vi "Hardware Config.vi"() -> ()   [LabVIEW 2022 SP3]
uses:
  Controls/Config.ctl
panel:
  in  "Signal list":bool
  out "Config":T1={"AO config"=[], "AI config"=[], "DI config"=[], "DO config"=[], "TC config"=[{"Channel_Name"="", "Channel_Number"="", "Pre_Scale_min"=0.0, "Pre_Scale_max"=0.0, "units"=4, " type"=7}], "ACC config"=[], "SG config"=[], "Strain Gauge Settings"={"poisson ratio"=0.3, "nominal gage resistance"=120.0, "gage factor"=2.08}, "Bridge Settings"={"voltage excitation value"=3.3, "voltage excitation source"=10200, "initial bridge voltage"=0.0, "lead wire resistance"=1.7, "strain configuration"=10271}, "Sample Rate"={"AI Sample Rate"=[], "AO Sample Rate"=[], "DI Sample Rate"=[], "TC Sample Rate"=[], "DO Sample Rate"=[], "SG Sample Rate"=[], "ACC Sample Rate"=[]}} {"Bridge Settings"."strain configuration" items=["Full Bridge I"=10183, "Full Bridge II"=10184, "Full Bridge III"=10185, "Half Bridge I"=10188, "Half Bridge II"=10189, "Quarter Bridge I"=10271, "Quarter Bridge II"=10272]; "Bridge Settings"."voltage excitation source" items=["Internal"=10200, "External"=10167, "None"=10230]; "ACC config"."Terminal configuration" items=["default"=-1, "RSE"=10083, "NRSE"=10078, "Differential"=10106, "Pseudodifferential"=12529]; "ACC config"."Sensitivity units" items=["mVolts/g"=12509, "Volts/g"=12510]; "TC config"."type" items=["J"=10072, "K"=10073, "N"=10077, "R"=10082, "S"=10085, "T"=10086, "B"=10047, "E"=10055]; "TC config"."units" items=["Deg C", "Deg F", "Kelvins", "Deg R", "From Custom Scale"]}
  in  "Cancel":bool
  in  "Load Configuration":bool
  in  "New configuration":bool
  in  "Save Config":bool
  in  "Tab Control":T2(tab)
  in  "DO Sample Rate":dbl[](array[numeric]) format="%#_g Hz"
  in  "DO config":T3(array[cluster])=[{"Channel_Name"="", "Channel_Number"="", "Default_Value"=FALSE, "Units"=FALSE}]
  out "DO Device List":string[](array[string])
  in  "DI Sample Rate":dbl[](array[numeric]) format="%#_g Hz"
  in  "DI config":T3(array[cluster])
  out "DI Device List":string[](array[string])
  in  "AO Sample Rate":dbl[](array[numeric]) format="%#_g Hz"
  in  "AO config":T4(array[cluster])
  out "AO Device List":string[](array[string])
  in  "AI Sample Rate":dbl[](array[numeric]) format="%#_g Hz"
  in  "AI config":T5(array[cluster])
  out "AI Device List":string[](array[string])
  in  "TC Sample Rate":dbl[](array[numeric]) format="%#_g Hz"
  in  "TC config":T6(array[cluster]) {"thermocouple type" items=["J", "K", "N", "R", "S", "T", "B", "E"]; "units" items=["Deg C", "Deg F", "Kelvins", "Deg R", "From Custom Scale"]}
  out "TC Device List":string[](array[string])
  in  "ACC Sample Rate":dbl[](array[numeric]) format="%#_g Hz"
  in  "ACC config":T7(array[cluster]) {"Sensitivity units" items=["mVolts/g"=12509, "Volts/g"=12510]; "Terminal configuration" items=["default"=-1, "RSE"=10083, "NRSE"=10078, "Differential"=10106, "Pseudodifferential"=12529]}
  out "ACC Device List":string[](array[string])
  out "SG Device List":string[](array[string])
  in  "SG Sample Rate":dbl[](array[numeric]) format="%#_g Hz"
  in  "SG config":T8(array[cluster])
  in  "SG Settings":T9={"gage factor"=2.08, "nominal gage \nresistance"=120.0, "poisson ratio"=0.3}
  in  "Bridge Settings":T10={"voltage excitation value"=3.3, "voltage excitation source"=10200, "initial bridge voltage"=0.0, "lead wire resistance"=1.7, "strain configuration"=10271} {"strain configuration" items=["Full Bridge I"=10183, "Full Bridge II"=10184, "Full Bridge III"=10185, "Half Bridge I"=10188, "Half Bridge II"=10189, "Quarter Bridge I"=10271, "Quarter Bridge II"=10272]; "voltage excitation source" items=["Internal"=10200, "External"=10167, "None"=10230]}
  # "DO_Channel_Name"
  # "DO_Channel_Number"
  # "Default Value"
  # "Invert?"
  # "DI_Channel_Name"
  # "DI_Channel_Number"
  # "Default Value"
  # "Invert?"
  # "AO_Channel_Name"
  # "AO_Channel_Number"
  # "Default Value"
  # "Units"
  # "AI_Channel_Name"
  # "AI_Channel_Number"
  # "Pre_Scale_min"
  # "Pre_Scale_max"
  # "Scale_min"
  # "Scale_max"
  # "Units"
  # "TC_Channel_Name"
  # "TC_Channel_Number"
  # "Max_Value"
  # "Units"
  # "Type"
  # "Min_Value"
  # "ACC_Channel_Name"
  # "ACC_Channel_Number"
  # "Min_Value"
  # "Max_Value"
  # "Terminal Config"
  # "Sensitivity"
  # "Sensitivity Units"
  # "SG_Channel_Name"
  # "SG_Channel_Number"
  # "Min_Value"
  # "Max_Value"
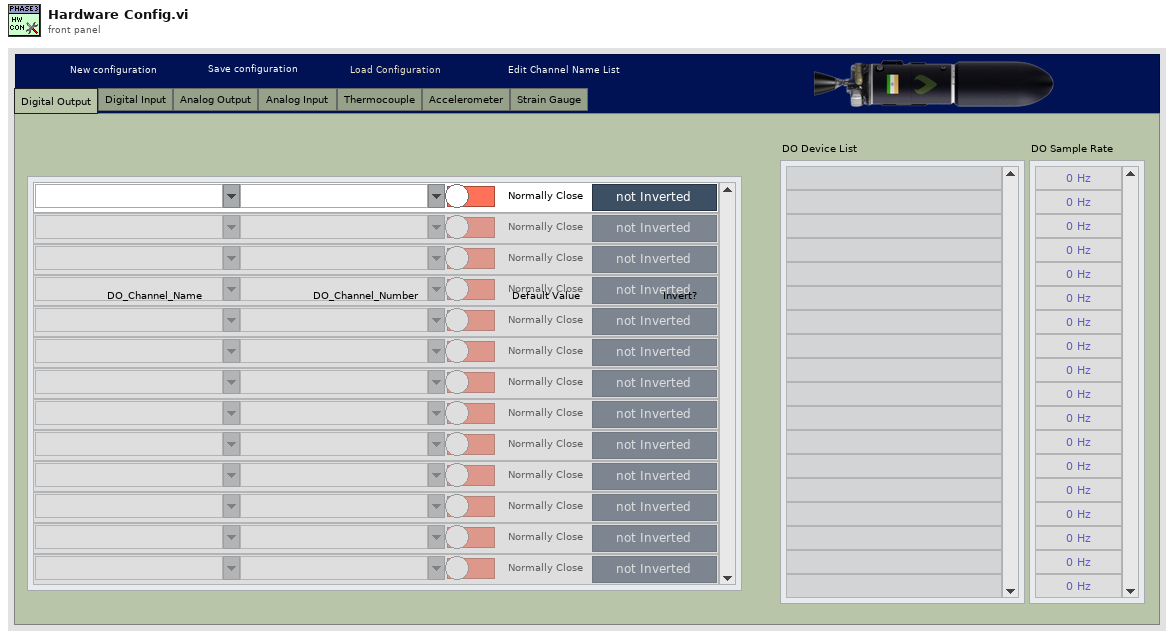
[diagram p1: front panel]
types:
  T1 = typedef "Config.ctl" = cluster{"AO config":cluster{"Channel_Name":string, "Channel_Number":string, "Default_Value":dbl, "Units":string}[], "AI config":cluster{"Channel_Name":string, "Channel_Number":string, "Pre_Scale_min":dbl, "Pre_Scale_max":dbl, "Sensor_min":dbl, "Sensor_max":dbl, "Units":string}[], "DI config":cluster{"Channel_Name":string, "Channel_Number":string, "Default_Value":bool, "DI invert?":bool}[], "DO config":cluster{"Channel_Name":string, "Channel_Number":string, "Default_Value":bool, "DO invert?":bool}[], "TC config":cluster{"Channel_Name":string, "Channel_Number":string, "Pre_Scale_min":dbl, "Pre_Scale_max":dbl, "units":i32, " type":i32}[], "ACC config":cluster{"Channel_Name":string, "Channel_Number":string, "Pre_Scale_min":dbl, "Pre_Scale_max":dbl, "Terminal configuration":i32, "Sensitivity":dbl, "Sensitivity units":i32}[], "SG config":cluster{"Channel_Name":string, "Channel_Number":string, "Pre_Scale_min":dbl, "Pre_Scale_max":dbl}[], "Strain Gauge Settings":cluster{"poisson ratio":dbl, "nominal gage resistance":dbl, "gage factor":dbl}, "Bridge Settings":cluster{"voltage excitation value":dbl, "voltage excitation source":i32, "initial bridge voltage":dbl, "lead wire resistance":dbl, "strain configuration":i32}, "Sample Rate":cluster{"AI Sample Rate":dbl[], "AO Sample Rate":dbl[], "DI Sample Rate":dbl[], "TC Sample Rate":dbl[], "DO Sample Rate":dbl[], "SG Sample Rate":dbl[], "ACC Sample Rate":dbl[]}}
  T2 = enum32{"Digital Output", "Digital Input", "Analog Output", "Analog Input ", "Thermocouple", "Accelerometer", "Strain Gauge"}
  T3 = cluster{"Channel_Name":string, "Channel_Number":string, "Default_Value":bool, "Units":bool}[]
  T4 = cluster{"Channel_Name":string, "Channel_Number":string, "Default_Value":dbl, "Units":string}[]
  T5 = cluster{"Channel_Name":string, "Channel_Number":string, "Pre_Scale_min":dbl, "Pre_Scale_max":dbl, "Sensor_min":dbl, "Sensor_max":dbl, "Units":string}[]
  T6 = cluster{"Channel_Name":string, "Channel_Number":string, "Pre_Scale_min":dbl, "Pre_Scale_max":dbl, "units":i32, "thermocouple type":i32}[]
  T7 = cluster{"Channel_Name":string, "Channel_Number":string, "Pre_Scale_min":dbl, "Pre_Scale_max":dbl, "Terminal configuration":i32, "Sensitivity":dbl, "Sensitivity units":i32}[]
  T8 = cluster{"Channel_Name":string, "Channel_Number":string, "Pre_Scale_min":dbl, "Pre_Scale_max":dbl}[]
  T9 = cluster{"gage factor":dbl, "nominal gage \nresistance":dbl, "poisson ratio":dbl}
  T10 = cluster{"voltage excitation value":dbl, "voltage excitation source":i32, "initial bridge voltage":dbl, "lead wire resistance":dbl, "strain configuration":i32}
  T11 = cluster{"Data":T1, "path":path, "Name ref":refnum<vi>[], "Names":string[][], "Signal path":path, "SR":cluster{"AI Sample Rate":dbl[], "AO Sample Rate":dbl[], "DI Sample Rate":dbl[], "TC Sample Rate":dbl[], "DO Sample Rate":dbl[], "SG Sample Rate":dbl[], "ACC Sample Rate":dbl[]}, "Device List":cluster{"AO Cards":tag[], "AI Cards":tag[], "DI Cards":tag[], "DO Cards":tag[]}}
  T12 = typedef "file folder ctl.ctl" = cluster{"Datalog path":path, "Configuration path":path, "Signal list path":path, "Sub vi's":path, "Authentication":path}
  T13 = cluster{"AI":string[], "DI":string[], "DO":string[], "SG":string[], "AO":string[], "TC":string[], "ACC":string[]}
  T14 = cluster{"AO Cards":tag[], "AI Cards":tag[], "DI Cards":tag[], "DO Cards":tag[]}
  T15 = cluster{"AI Channel list":tag[], "AO Channel list":tag[], "DO Channel list ":tag[], "DI Channel list":tag[]}
  T16 = cluster{"AI Sample Rate":dbl[], "AO Sample Rate":dbl[], "DI Sample Rate":dbl[], "TC Sample Rate":dbl[], "DO Sample Rate":dbl[], "SG Sample Rate":dbl[], "ACC Sample Rate":dbl[]}
  T17 = enum16{"open", "replace", "create", "open or create", "replace or create", "replace or create with confirmation"}
  T18 = enum32{"Invalid", "Standard", "Closed", "Hidden", "Minimized", "Maximized"}
  T19 = cluster{"Channel_Name":string, "Channel_Number":string, "Default_Value":bool, "DI invert?":bool}[]
  T20 = cluster{"Channel_Name":string, "Channel_Number":string, "Default_Value":bool, "DO invert?":bool}[]
  T21 = cluster{"Channel_Name":string, "Channel_Number":string, "Pre_Scale_min":dbl, "Pre_Scale_max":dbl, "units":i32, " type":i32}[]
  T22 = cluster{"poisson ratio":dbl, "nominal gage resistance":dbl, "gage factor":dbl}
  T23 = cluster{"Channel_Name":string, "Channel_Number":string}
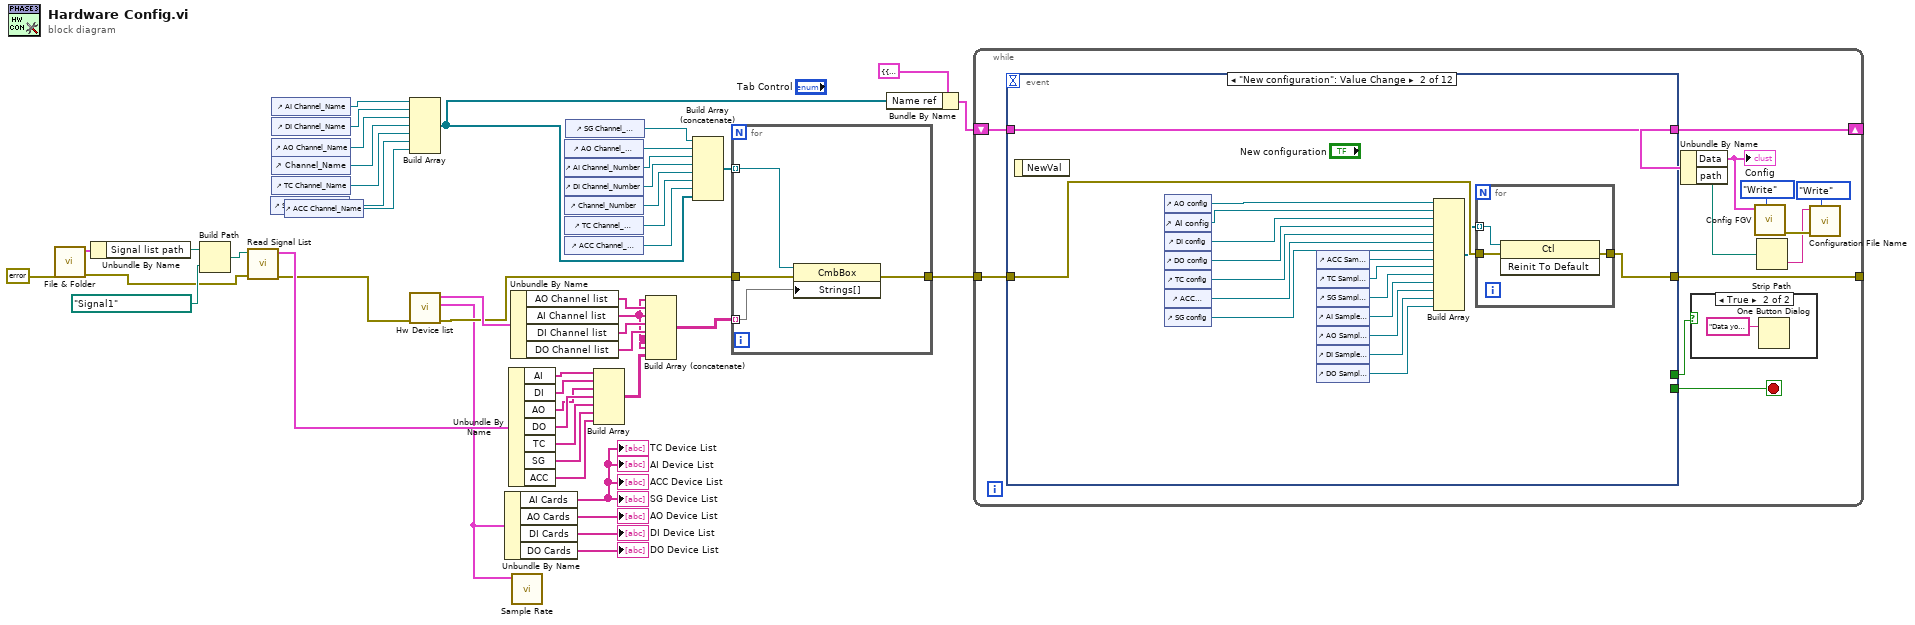
[diagram p0: block diagram]
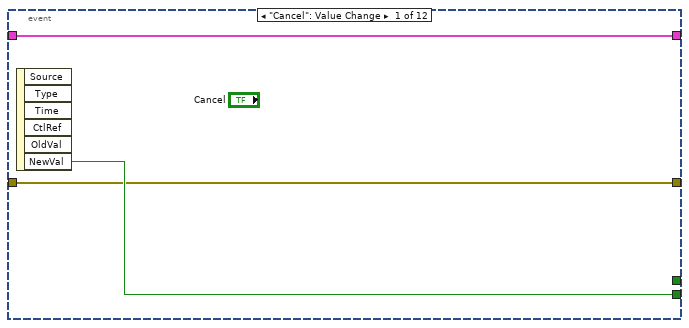
[diagram p3: hidden frame]
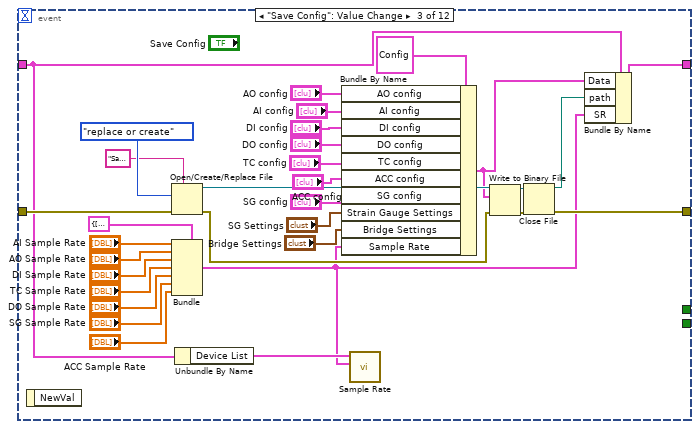
[diagram p4: hidden frame]
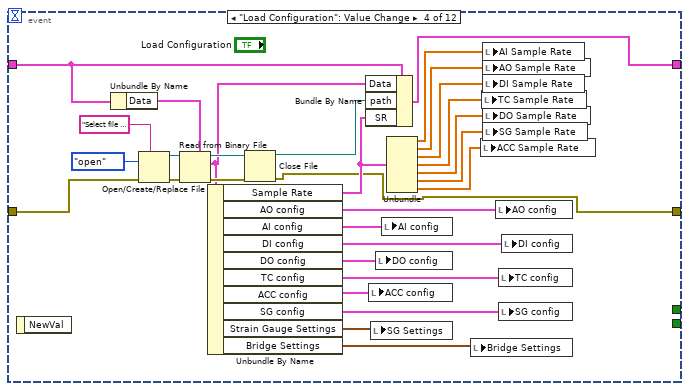
[diagram p5: hidden frame]
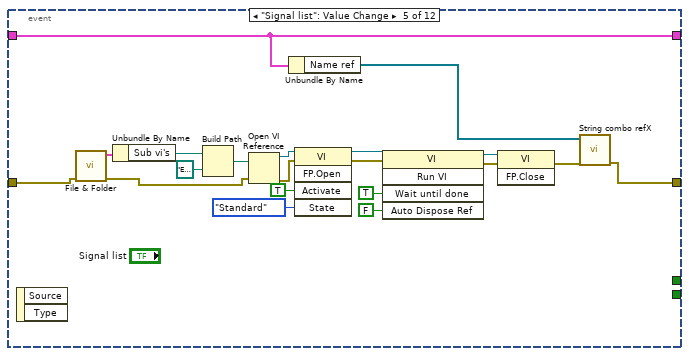
[diagram p6: hidden frame]
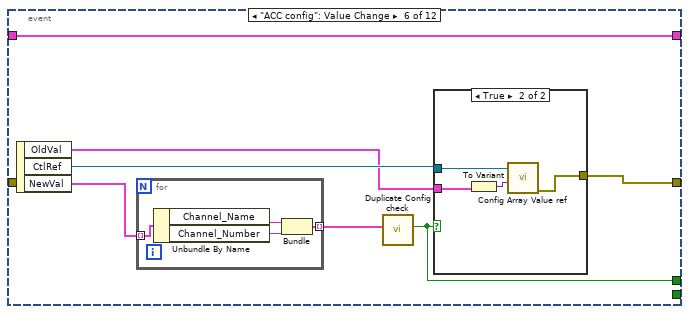
[diagram p7: hidden frame]
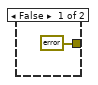
[diagram p8: hidden frame]
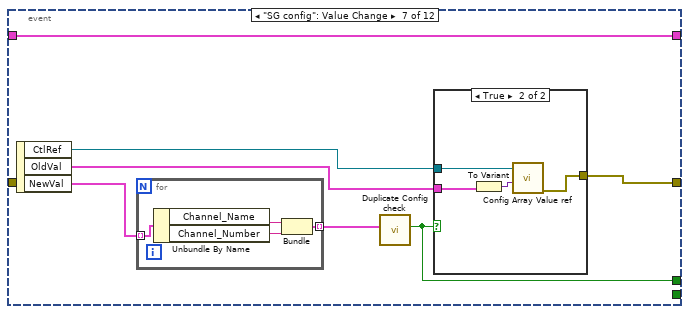
[diagram p9: hidden frame]
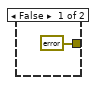
[diagram p10: hidden frame]
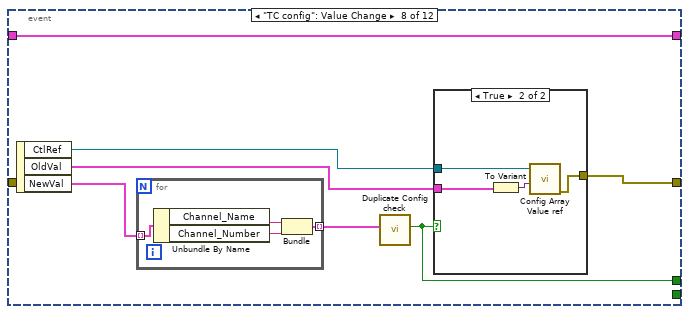
[diagram p11: hidden frame]
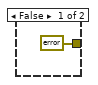
[diagram p12: hidden frame]
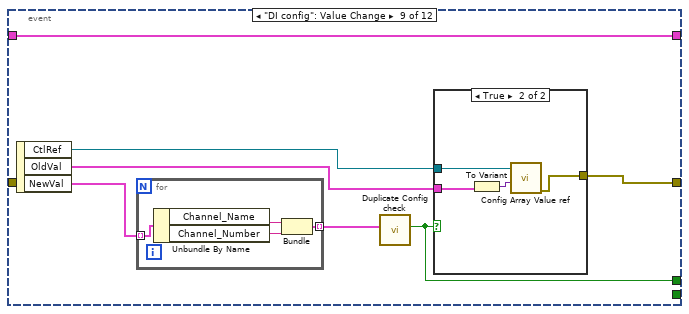
[diagram p13: hidden frame]
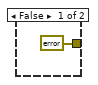
[diagram p14: hidden frame]
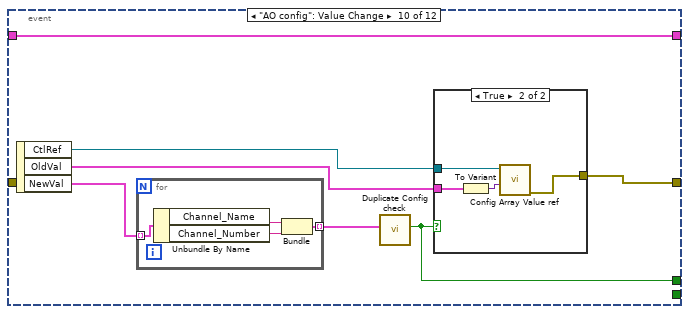
[diagram p15: hidden frame]
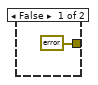
[diagram p16: hidden frame]
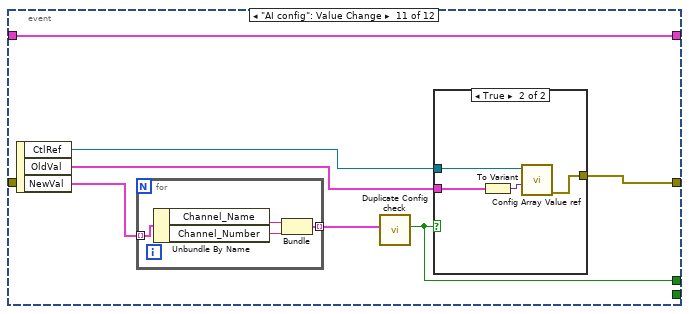
[diagram p17: hidden frame]
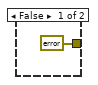
[diagram p18: hidden frame]
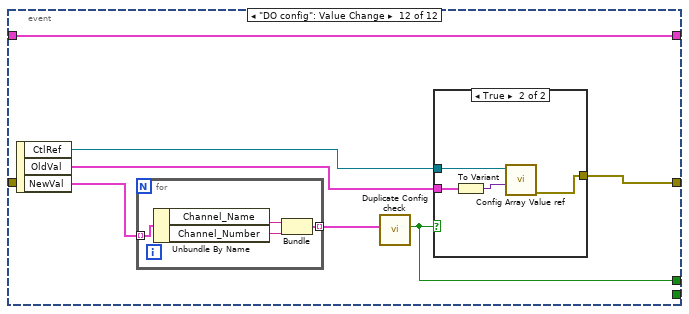
[diagram p19: hidden frame]
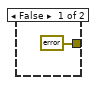
[diagram p20: hidden frame]
diagram:
  n1 = call "File & Folder.vi"("error in (no error)"=errorcluster {"status"=FALSE, "code"=0, "source"=""} ("error in")) -> ("error out"=w24:errorcluster, "File Output"=w30:T12)  [unwired: 9 in]
  n2 = Unbundle By Name(w30) -> ("Signal list path"=w29:path)
  n3 = Build Path(base path=w29, name or relative path=path "Signal1") -> (appended path=w1:path)
  n4 = call "Read Signal List.vi"("error in"=w24, "file path (use dialog)"=w1) -> ("error out"=w4:errorcluster, "Names"=w23:T13)  [unwired: 8 in]
  n5 = control-ref of="SG Channel_Name"() -> (w9:refnum<vi>)
  n6 = control-ref of="AI Channel_Name"() -> (w27:refnum<vi>)
  n7 = control-ref of="DI Channel_Name"() -> (w26:refnum<vi>)
  n8 = control-ref of="AO Channel_Name"() -> (w11:refnum<vi>)
  n9 = control-ref of="Channel_Name"() -> (w10:refnum<vi>)
  n10 = control-ref of="TC Channel_Name"() -> (w25:refnum<vi>)
  n11 = control-ref of="ACC Channel_Name"() -> (w8:refnum<vi>)
  n12 = Build Array(w27, w26, w11, w10, w25, w9, w8) -> (w12:refnum<vi>[])
  n13 = call "Hw Device list.vi"("error in (no error)"=w4) -> ("error out"=w38:errorcluster, "Device List"=w2:T14, "Channel List"=w39:T15)  [unwired: 8 in]
  n14 = Unbundle By Name(w2) -> ("AI Cards"=→"AI Device List" →"TC Device List" →"ACC Device List" →"SG Device List":tag[], "AO Cards"=→"AO Device List":tag[], "DI Cards"=→"DI Device List":tag[], "DO Cards"=→"DO Device List":tag[])
  n15 = Unbundle By Name(w23) -> ("AI"=w22:string[], "DI"=w21:string[], "AO"=w16:string[], "DO"=w20:string[], "TC"=w19:string[], "SG"=w18:string[], "ACC"=w17:string[])
  n16 = Unbundle By Name(w39) -> ("AO Channel list"=w33:tag[], "AI Channel list"=w32:tag[], "DI Channel list"=w42:tag[], "DO Channel list"=w41:tag[])
  n17 = call "Sample Rate.vi"("Device List"=w2) -> ()  [unwired: 11 in]
  n18 = control-ref of="AO Channel_Number"() -> (w47:refnum<vi>)
  n19 = control-ref of="AI Channel_Number"() -> (w46:refnum<vi>)
  n20 = control-ref of="DI Channel_Number"() -> (w45:refnum<vi>)
  n21 = control-ref of="Channel_Number"() -> (w44:refnum<vi>)
  n22 = control-ref of="TC Channel_Number"() -> (w36:refnum<vi>)
  n23 = control-ref of="ACC Channel_Number"() -> (w35:refnum<vi>)
  n24 = control-ref of="SG Channel_Number"() -> (w34:refnum<vi>)
  n25 = Build Array(w22, w21, w16, w20, w19, w18, w17) -> (w15:string[][])
  n26 = Build Array (concatenate)(w32, w33, w32, w42, w41, w32, w32, w15) -> (w40:string[][])
  n27 = Build Array (concatenate)(w34, w47, w46, w45, w44, w36, w35, w12) -> (w43:refnum<vi>[])
  n28 = for {
    tunnel: w43 -> [w51] mode=indexing
    tunnel: w40 -> [w48] mode=indexing
    tunnel: [w50] -> w37
    tunnel: w38 -> [w49]
    n29 = property class="CmbBox"(reference=w51, error in=w49, "Strings[]"=w48) -> (error out=w50:errorcluster)  [unwired: 1 out]
  }
  n30 = Bundle By Name(cluster=T11 {"Data"={"AO config"=[], "AI config"=[], "DI config"=[], "DO config"=[], "TC config"=[{"Channel_Name"="", "Channel_Number"="", "Pre_Scale_min"=0.0, "Pre_Scale_max"=0.0, "units"=4, " type"=7}], "ACC config"=[], "SG config"=[], "Strain Gauge Settings"={"poisson ratio"=0.3, "nominal gage resistance"=120.0, "gage factor"=2.08}, "Bridge Settings"={"voltage excitation value"=3.3, "voltage excitation source"=10200, "initial bridge voltage"=0.0, "lead wire resistance"=1.7, "strain configuration"=10271}, "Sample Rate"={"AI Sample Rate"=[], "AO Sample Rate"=[], "DI Sample Rate"=[], "TC Sample Rate"=[], "DO Sample Rate"=[], "SG Sample Rate"=[], "ACC Sample Rate"=[]}}, "path"=path "", "Name ref"=[], "Names"=[], "Signal path"=path "", "SR"={"AI Sample Rate"=[], "AO Sample Rate"=[], "DI Sample Rate"=[], "TC Sample Rate"=[], "DO Sample Rate"=[], "SG Sample Rate"=[], "ACC Sample Rate"=[]}, "Device List"={"AO Cards"=["PXI1Slot2"], "AI Cards"=["cDAQ1Mod1", "cDAQ1Mod2", "cDAQ1Mod3", "cDAQ1Mod4"], "DI Cards"=["cDAQ1Mod5", "PXI1Slot2", "PXI1Slot3"], "DO Cards"=["cDAQ1Mod5", "PXI1Slot2", "PXI1Slot3"]}}, "Name ref"=w12) -> (w14:T11)
  n31 = while {
    shift-right: [w59] -> _
    shift-left: w14 -> [w60]
    tunnel: w37 -> [w62]
    tunnel: [w61] -> _
    stop <- w63 stop-if-true
    n32 = event shown="[1] \"New configuration\": Value Change" {
      selector: _ -> [_ _ _ _ _ _ _ _ _ _ _ _]
      dyn-events: _ -> [_ _ _ _ _ _ _ _ _ _ _ _]
      timeout: _ -> [_ _ _ _ _ _ _ _ _ _ _ _]
      tunnel: [w66 _ _ _ _ _ _ _ _ _ _ _] -> w63
      tunnel: w62 -> [w65 w85 w120 w150 w170 _ _ _ _ _ _ _]
      tunnel: [w65 w84 w116 w127 w152 w172 w190 w206 w222 w238 w254 w270] -> w61
      tunnel: w60 -> [w67 w83 w91 w141 w155 w177 w193 w209 w225 w241 w257 w273]
      tunnel: [w67 w83 w108 w142 w155 w177 w193 w209 w225 w241 w257 w273] -> w59
      tunnel: [_ _ _ _ _ w171 w187 w203 w219 w235 w251 w267] -> w55
      event "Cancel": Value Change {
        n33 = event-data() -> ("NewVal"=w66:bool)  [unwired: 1 in, 5 out]
      }
      event "New configuration": Value Change {
        n34 = event-data() -> ()  [unwired: 1 in, 1 out]
        n35 = control-ref of="AO config"() -> (w78:refnum<vi>)
        n36 = control-ref of="AI config"() -> (w79:refnum<vi>)
        n37 = control-ref of="DI config"() -> (w80:refnum<vi>)
        n38 = control-ref of="DO config"() -> (w81:refnum<vi>)
        n39 = control-ref of="TC config"() -> (w77:refnum<vi>)
        n40 = control-ref of="ACC config"() -> (w76:refnum<vi>)
        n41 = control-ref of="SG config"() -> (w75:refnum<vi>)
        n42 = control-ref of="ACC Sample Rate"() -> (w74:refnum<vi>)
        n43 = control-ref of="TC Sample Rate"() -> (w73:refnum<vi>)
        n44 = control-ref of="SG Sample Rate"() -> (w72:refnum<vi>)
        n45 = control-ref of="AI Sample Rate"() -> (w71:refnum<vi>)
        n46 = control-ref of="AO Sample Rate"() -> (w70:refnum<vi>)
        n47 = control-ref of="DI Sample Rate"() -> (w69:refnum<vi>)
        n48 = control-ref of="DO Sample Rate"() -> (w68:refnum<vi>)
        n49 = Build Array(w78, w79, w80, w81, w77, w76, w75, w74, w73, w72, w71, w70, w69, w68) -> (w82:refnum<vi>[])
        n50 = for {
          tunnel: w82 -> [w88] mode=indexing
          tunnel: w85 -> [w87]
          tunnel: [w86] -> w84
          n51 = invoke class="Ctl" method="Reinit To Default"(reference=w88, error in=w87) -> (error out=w86:errorcluster)  [unwired: 1 in, 2 out]
        }
      }
      event "Save Config": Value Change {
        n52 = event-data() -> ()  [unwired: 1 in, 1 out]
        n53 = Open/Create/Replace File(error in=w120, prompt="Save Changes", operation (0:open)=T17."replace or create") -> (refnum out=w115:refnum<file>, error out=w119:errorcluster)  [unwired: 3 in, 1 out]
        n54 = Bundle(cluster=T16 {"AI Sample Rate"=[], "AO Sample Rate"=[], "DI Sample Rate"=[], "TC Sample Rate"=[], "DO Sample Rate"=[], "SG Sample Rate"=[], "ACC Sample Rate"=[]} ("Sample Rate"), "AI Sample Rate"="AI Sample Rate", "AO Sample Rate"="AO Sample Rate", "DI Sample Rate"="DI Sample Rate", "TC Sample Rate"="TC Sample Rate", "DO Sample Rate"="DO Sample Rate", "SG Sample Rate"="SG Sample Rate", "ACC Sample Rate"="ACC Sample Rate") -> (w89:T16)
        n55 = Unbundle By Name(w91) -> ("Device List"=w90:T14)
        n56 = Bundle By Name(cluster=T1 {"AO config"=[], "AI config"=[], "DI config"=[], "DO config"=[], "TC config"=[{"Channel_Name"="", "Channel_Number"="", "Pre_Scale_min"=0.0, "Pre_Scale_max"=0.0, "units"=4, " type"=7}], "ACC config"=[], "SG config"=[], "Strain Gauge Settings"={"poisson ratio"=0.3, "nominal gage resistance"=120.0, "gage factor"=2.08}, "Bridge Settings"={"voltage excitation value"=3.3, "voltage excitation source"=10200, "initial bridge voltage"=0.0, "lead wire resistance"=1.7, "strain configuration"=10271}, "Sample Rate"={"AI Sample Rate"=[], "AO Sample Rate"=[], "DI Sample Rate"=[], "TC Sample Rate"=[], "DO Sample Rate"=[], "SG Sample Rate"=[], "ACC Sample Rate"=[]}} ("Data"), "AO config"="AO config", "AI config"="AI config", "DI config"="DI config", "DO config"="DO config", "TC config"="TC config", "ACC config"="ACC config", "SG config"="SG config", "Strain Gauge Settings"="SG Settings", "Bridge Settings"="Bridge Settings", "Sample Rate"=w89) -> (w106:T1)
        n57 = call "Sample Rate.vi"("Sample Rate"=w89, "Device List"=w90) -> ()  [unwired: 10 in]
        n58 = Write to Binary File(file (use dialog)=w115, data=w106, error in=w119) -> (refnum out=w118:refnum<file>, error out=w117:errorcluster)  [unwired: 3 in, 1 out]
        n59 = Close File(refnum=w118, error in=w117) -> (path=w102:path, error out=w116:errorcluster)
        n60 = Bundle By Name(cluster=w91, "Data"=w106, "path"=w102, "SR"=w89) -> (w108:T11)
      }
      event "Load Configuration": Value Change {
        n61 = event-data() -> ()  [unwired: 1 in, 1 out]
        n62 = Unbundle By Name(w141) -> ("Data"=w143:T1)
        n63 = Open/Create/Replace File(error in=w150, prompt="Select file to load", operation (0:open)=T17."open") -> (refnum out=w146:refnum<file>, error out=w149:errorcluster)  [unwired: 3 in, 1 out]
        n64 = Read from Binary File(5:w143, 8:w149, 11:w146) -> (0:w147:errorcluster, 2:w140:T1, 3:w148:refnum<file>)  [unwired: 3 in, 1 out]
        n65 = Unbundle By Name(w140) -> ("Sample Rate"=w129:T16, "AO config"=w139:T4, "AI config"=w138:T5, "DI config"=w137:T19, "DO config"=w136:T20, "TC config"=w135:T21, "ACC config"=w134:T7, "SG config"=w133:T8, "Strain Gauge Settings"=w131:T22, "Bridge Settings"=w130:T10)
        n66 = Close File(refnum=w148, error in=w147) -> (path=w132:path, error out=w127:errorcluster)
        n67 = Bundle By Name(cluster=w141, "Data"=w140, "path"=w132, "SR"=w129) -> (w142:T11)
        n68 = local write "ACC config"(w134) -> ()
        n69 = local write "SG Settings"(w131) -> ()
        n70 = local write "DO config"(w136) -> ()
        n71 = local write "AI config"(w138) -> ()
        n72 = Unbundle(w129) -> ("AI Sample Rate"=w128:dbl[], "AO Sample Rate"=w126:dbl[], "DI Sample Rate"=w125:dbl[], "TC Sample Rate"=w124:dbl[], "DO Sample Rate"=w123:dbl[], "SG Sample Rate"=w122:dbl[], "ACC Sample Rate"=w121:dbl[])
        n73 = local write "Bridge Settings"(w130) -> ()
        n74 = local write "ACC Sample Rate"(w121) -> ()
        n75 = local write "TC Sample Rate"(w124) -> ()
        n76 = local write "AI Sample Rate"(w128) -> ()
        n77 = local write "AO Sample Rate"(w126) -> ()
        n78 = local write "DI Sample Rate"(w125) -> ()
        n79 = local write "DO Sample Rate"(w123) -> ()
        n80 = local write "SG Sample Rate"(w122) -> ()
        n81 = local write "AO config"(w139) -> ()
        n82 = local write "TC config"(w135) -> ()
        n83 = local write "SG config"(w133) -> ()
        n84 = local write "DI config"(w137) -> ()
      }
      event "Signal list": Value Change {
        n85 = event-data() -> ()  [unwired: 1 in, 2 out]
        n86 = call "File & Folder.vi"("error in (no error)"=w170) -> ("error out"=w166:errorcluster, "File Output"=w169:T12)  [unwired: 9 in]
        n87 = Unbundle By Name(w169) -> ("Sub vi's"=w168:path)
        n88 = Build Path(base path=w168, name or relative path=path "Edit Channel Name list.vi") -> (appended path=w151:path)
        n89 = Open VI Reference(vi path=w151, error in (no error)=w166) -> (vi reference=w157:refnum<vi>, error out=w156:errorcluster)  [unwired: 4 in]
        n90 = Unbundle By Name(w155) -> ("Name ref"=w154:refnum<vi>[])
        n91 = invoke class="VI" method="FP.Open"(reference=w157, error in=w156, "Activate"=TRUE ("Activate?"), "State"=T18."Standard") -> (reference out=w165:refnum<vi>, error out=w164:errorcluster)  [unwired: 1 in, 3 out]
        n92 = invoke class="VI" method="Run VI"(reference=w165, error in=w164, "Wait until done"=TRUE ("Wait Until Done"), "Auto Dispose Ref"=FALSE ("Auto Dispose Reference")) -> (reference out=w163:refnum<vi>, error out=w162:errorcluster)  [unwired: 1 in, 3 out]
        n93 = invoke class="VI" method="FP.Close"(reference=w163, error in=w162) -> (error out=w153:errorcluster)  [unwired: 1 in, 2 out]
        n94 = call "String combo refX.vi"("error out"=w153, "Ctrl ref"=w154) -> ("error out 2"=w152:errorcluster)  [unwired: 9 in]
      }
      event "ACC config": Value Change {
        n95 = event-data() -> ("OldVal"=w173:T7, "CtlRef"=w174:refnum<vi>, "NewVal"=w176:T7)  [unwired: 1 in]
        n96 = for {
          tunnel: w176 -> [w181] mode=indexing
          tunnel: [w178] -> w175 mode=indexing
          n97 = Unbundle By Name(w181) -> ("Channel_Name"=w179:string, "Channel_Number"=w180:string)
          n98 = Bundle("Channel_Name"=w179, "Channel_Number"=w180) -> (w178:T23)  [unwired: 1 in]
        }
        n99 = call "Duplicate Config check.vi"("Data in"=w175) -> ("Channel list indication"=w171:bool)  [unwired: 10 in]
        n100 = case shown="True" w171 {
          tunnel: w174 -> [_ w185]
          tunnel: w173 -> [_ w184]
          tunnel: [errorcluster {"status"=FALSE, "code"=0, "source"=""} ("error out") w183] -> w172
          frame False {
          }
          frame True {
            n101 = To Variant(anything=w184) -> (Variant=w186:variant)
            n102 = call "Config Array Value ref.vi"("Value"=w186, "Array in"=w185) -> ("error out"=w183:errorcluster)  [unwired: 9 in]
          }
        }
      }
      event "SG config": Value Change {
        n103 = event-data() -> ("CtlRef"=w189:refnum<vi>, "OldVal"=w188:T8, "NewVal"=w192:T8)  [unwired: 1 in]
        n104 = for {
          tunnel: w192 -> [w197] mode=indexing
          tunnel: [w194] -> w191 mode=indexing
          n105 = Unbundle By Name(w197) -> ("Channel_Name"=w195:string, "Channel_Number"=w196:string)
          n106 = Bundle("Channel_Name"=w195, "Channel_Number"=w196) -> (w194:T23)  [unwired: 1 in]
        }
        n107 = call "Duplicate Config check.vi"("Data in"=w191) -> ("Channel list indication"=w187:bool)  [unwired: 10 in]
        n108 = case shown="True" w187 {
          tunnel: w189 -> [_ w201]
          tunnel: w188 -> [_ w200]
          tunnel: [errorcluster {"status"=FALSE, "code"=0, "source"=""} ("error out") w199] -> w190
          frame False {
          }
          frame True {
            n109 = To Variant(anything=w200) -> (Variant=w202:variant)
            n110 = call "Config Array Value ref.vi"("Value"=w202, "Array in"=w201) -> ("error out"=w199:errorcluster)  [unwired: 9 in]
          }
        }
      }
      event "TC config": Value Change {
        n111 = event-data() -> ("CtlRef"=w205:refnum<vi>, "OldVal"=w204:T6, "NewVal"=w208:T6)  [unwired: 1 in]
        n112 = for {
          tunnel: w208 -> [w213] mode=indexing
          tunnel: [w210] -> w207 mode=indexing
          n113 = Unbundle By Name(w213) -> ("Channel_Name"=w211:string, "Channel_Number"=w212:string)
          n114 = Bundle("Channel_Name"=w211, "Channel_Number"=w212) -> (w210:T23)  [unwired: 1 in]
        }
        n115 = call "Duplicate Config check.vi"("Data in"=w207) -> ("Channel list indication"=w203:bool)  [unwired: 10 in]
        n116 = case shown="True" w203 {
          tunnel: w205 -> [_ w217]
          tunnel: w204 -> [_ w216]
          tunnel: [errorcluster {"status"=FALSE, "code"=0, "source"=""} ("error out") w215] -> w206
          frame False {
          }
          frame True {
            n117 = To Variant(anything=w216) -> (Variant=w218:variant)
            n118 = call "Config Array Value ref.vi"("Value"=w218, "Array in"=w217) -> ("error out"=w215:errorcluster)  [unwired: 9 in]
          }
        }
      }
      event "DI config": Value Change {
        n119 = event-data() -> ("CtlRef"=w221:refnum<vi>, "OldVal"=w220:T3, "NewVal"=w224:T3)  [unwired: 1 in]
        n120 = for {
          tunnel: w224 -> [w229] mode=indexing
          tunnel: [w226] -> w223 mode=indexing
          n121 = Unbundle By Name(w229) -> ("Channel_Name"=w227:string, "Channel_Number"=w228:string)
          n122 = Bundle("Channel_Name"=w227, "Channel_Number"=w228) -> (w226:T23)  [unwired: 1 in]
        }
        n123 = call "Duplicate Config check.vi"("Data in"=w223) -> ("Channel list indication"=w219:bool)  [unwired: 10 in]
        n124 = case shown="True" w219 {
          tunnel: w221 -> [_ w233]
          tunnel: w220 -> [_ w232]
          tunnel: [errorcluster {"status"=FALSE, "code"=0, "source"=""} ("error out") w231] -> w222
          frame False {
          }
          frame True {
            n125 = To Variant(anything=w232) -> (Variant=w234:variant)
            n126 = call "Config Array Value ref.vi"("Value"=w234, "Array in"=w233) -> ("error out"=w231:errorcluster)  [unwired: 9 in]
          }
        }
      }
      event "AO config": Value Change {
        n127 = event-data() -> ("CtlRef"=w237:refnum<vi>, "OldVal"=w236:T4, "NewVal"=w240:T4)  [unwired: 1 in]
        n128 = for {
          tunnel: w240 -> [w245] mode=indexing
          tunnel: [w242] -> w239 mode=indexing
          n129 = Unbundle By Name(w245) -> ("Channel_Name"=w243:string, "Channel_Number"=w244:string)
          n130 = Bundle("Channel_Name"=w243, "Channel_Number"=w244) -> (w242:T23)  [unwired: 1 in]
        }
        n131 = call "Duplicate Config check.vi"("Data in"=w239) -> ("Channel list indication"=w235:bool)  [unwired: 10 in]
        n132 = case shown="True" w235 {
          tunnel: w237 -> [_ w250]
          tunnel: w236 -> [_ w248]
          tunnel: [errorcluster {"status"=FALSE, "code"=0, "source"=""} ("error out") w249] -> w238
          frame False {
          }
          frame True {
            n133 = To Variant(anything=w248) -> (Variant=w247:variant)
            n134 = call "Config Array Value ref.vi"("Value"=w247, "Array in"=w250) -> ("error out"=w249:errorcluster)  [unwired: 9 in]
          }
        }
      }
      event "AI config": Value Change {
        n135 = event-data() -> ("CtlRef"=w253:refnum<vi>, "OldVal"=w252:T5, "NewVal"=w256:T5)  [unwired: 1 in]
        n136 = for {
          tunnel: w256 -> [w261] mode=indexing
          tunnel: [w258] -> w255 mode=indexing
          n137 = Unbundle By Name(w261) -> ("Channel_Name"=w259:string, "Channel_Number"=w260:string)
          n138 = Bundle("Channel_Name"=w259, "Channel_Number"=w260) -> (w258:T23)  [unwired: 1 in]
        }
        n139 = call "Duplicate Config check.vi"("Data in"=w255) -> ("Channel list indication"=w251:bool)  [unwired: 10 in]
        n140 = case shown="True" w251 {
          tunnel: w253 -> [_ w265]
          tunnel: w252 -> [_ w264]
          tunnel: [errorcluster {"status"=FALSE, "code"=0, "source"=""} ("error out") w263] -> w254
          frame False {
          }
          frame True {
            n141 = To Variant(anything=w264) -> (Variant=w266:variant)
            n142 = call "Config Array Value ref.vi"("Value"=w266, "Array in"=w265) -> ("error out"=w263:errorcluster)  [unwired: 9 in]
          }
        }
      }
      event "DO config": Value Change {
        n143 = event-data() -> ("CtlRef"=w269:refnum<vi>, "OldVal"=w268:T3, "NewVal"=w272:T3)  [unwired: 1 in]
        n144 = for {
          tunnel: w272 -> [w277] mode=indexing
          tunnel: [w274] -> w271 mode=indexing
          n145 = Unbundle By Name(w277) -> ("Channel_Name"=w275:string, "Channel_Number"=w276:string)
          n146 = Bundle("Channel_Name"=w275, "Channel_Number"=w276) -> (w274:T23)  [unwired: 1 in]
        }
        n147 = call "Duplicate Config check.vi"("Data in"=w271) -> ("Channel list indication"=w267:bool)  [unwired: 10 in]
        n148 = case shown="True" w267 {
          tunnel: w269 -> [_ w282]
          tunnel: w268 -> [_ w280]
          tunnel: [errorcluster {"status"=FALSE, "code"=0, "source"=""} ("error out") w281] -> w270
          frame False {
          }
          frame True {
            n149 = To Variant(anything=w280) -> (Variant=w279:variant)
            n150 = call "Config Array Value ref.vi"("Value"=w279, "Array in"=w282) -> ("error out"=w281:errorcluster)  [unwired: 9 in]
          }
        }
      }
    }
    n151 = Unbundle By Name(w59) -> ("Data"=w58:T1, "path"=w56:path)
    "Config" <- w58
    n152 = case shown="True" w55 {
      frame False {
      }
      frame True {
        n153 = One Button Dialog ("Warning")(message="Data you Entered is already Exist!") -> ()  [unwired: 1 in, 1 out]
      }
    }
    n154 = call "Config FGV.vi"("Enum"=enum16{"Read", "Write"}."Write", "Data 2"=w58) -> ("error out"=w54:errorcluster)  [unwired: 8 in, 1 out]
    n155 = Strip Path(path=w56) -> (name=w53:string)  [unwired: 1 out]
    n156 = call "Configuration File Name.vi"("Enum"=enum16{"Read", "Write"}."Write", "error in"=w54, "Phase code W"=w53) -> ()  [unwired: 7 in, 2 out]
  }
